vi "parseLua.vi"() -> ()   [LabVIEW 2009, in "run.lvlib"]
uses:
  run.lvlib
panel:
  out "after":string
  out "before":string
  in  "Path":path
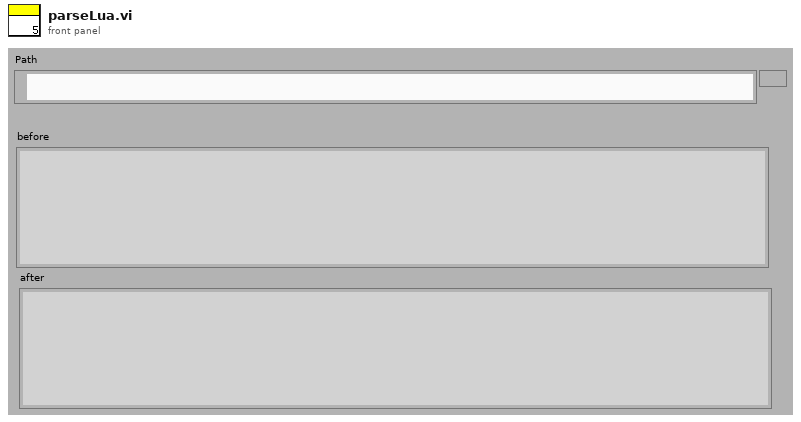
[diagram p1: front panel]
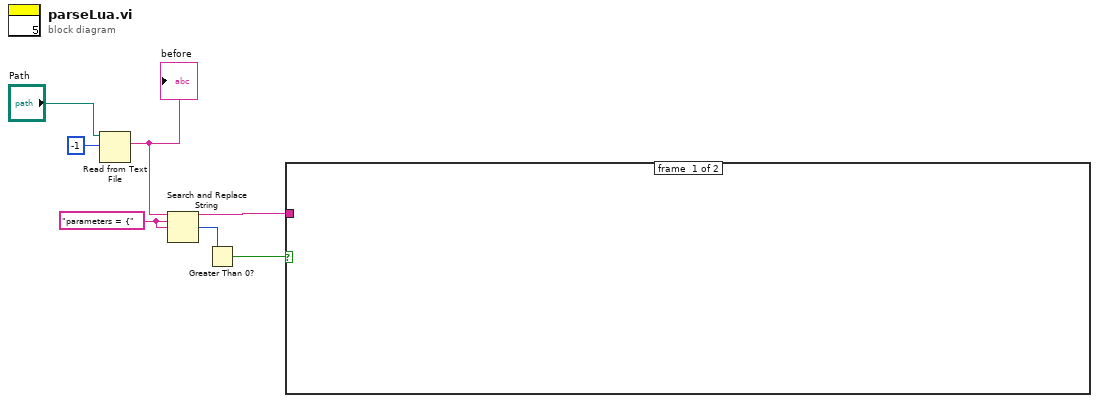
[diagram p0: block diagram]
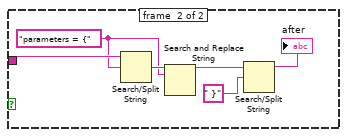
[diagram p2: hidden frame]
diagram:
  w1 = "parameters = {"
  n1 = Read from Text File(file (use dialog)="Path", count=-1) -> (text=w5:string)  [unwired: 2 in, 3 out]
  "before" <- w5
  n2 = Search and Replace String(input string=w5, search string=w1, replace string=w1) -> (result string=w2:string, number of replacements=w4:i32)  [unwired: 5 in, 2 out]
  n3 = Greater Than 0?(x=w4) -> (x > 0?=w3:bool)
  n4 = case shown="True" w3 {
    tunnel: w2 -> [_ w13]
    frame #0 {
    }
    frame #1 {
      w9 = "parameters = {"
      n5 = Search/Split String(string=w13, search string/char (-)=w9) -> (match + rest of string=w10:string)  [unwired: 1 in, 2 out]
      n6 = Search and Replace String(input string=w10, search string=w9) -> (result string=w8:string)  [unwired: 6 in, 3 out]
      n7 = Search/Split String(string=w8, search string/char (-)=" }") -> (substring before match=→"after":string)  [unwired: 1 in, 2 out]
    }
  }
